vi "Edit Poll.vi"(8 "error in (no error)":errorcluster, 11 "Node Ptr":u64 format="%.0x") -> (0 "error out":errorcluster)   [LabVIEW 2019, in "Diagnostics Addon System Explorer.lvlib"]
uses:
  Diagnostics Addon System Explorer.lvlib
  <vilib>/NI VeriStand/Custom Device Tools/Custom Device Utility Library/Custom Device Utility Library.lvlib
  Types/FG.Action.ctl
  <vilib>/NI VeriStand/Custom Device API/Custom Device API.lvlib
  Types/Poll.LinkedNode.ctl
panel:
  in  "Tag":string
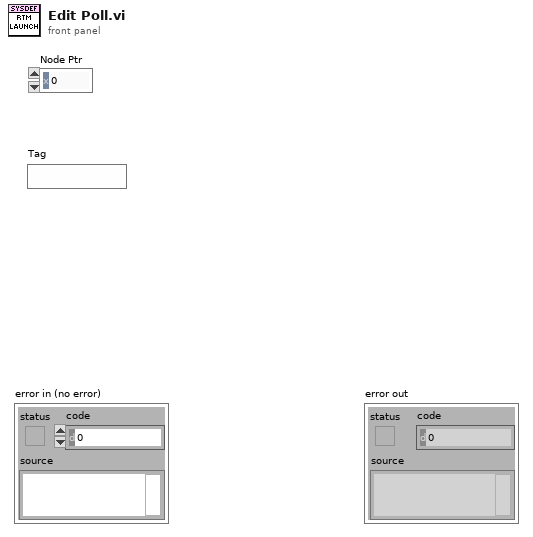
[diagram p1: front panel]
types:
  T1 = typedef "Diagnostics Addon System Explorer.lvlib/Poll.LinkedNode.ctl" = cluster{"Node ID":u64}
  T2 = typedef "Diagnostics Addon System Explorer.lvlib/FG.Action.ctl" = enum16{"Get", "Set"}
  T3 = typedef "Custom Device API.lvlib/Custom Device Item Ref.ctl" = u64
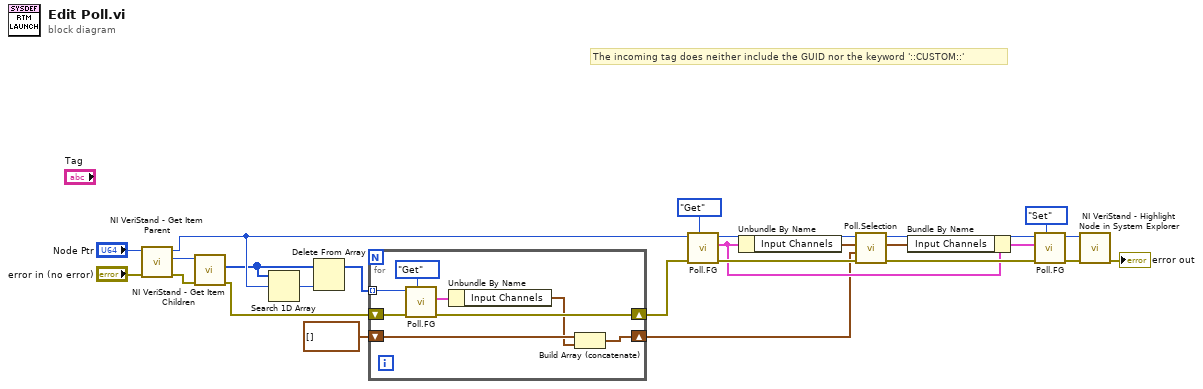
[diagram p0: block diagram]
diagram:
  # "The incoming tag does neither include the GUID nor the keyword '::CUSTOM::'"
  n1 = call <vilib>:"NI VeriStand - Get Item Parent.vi"("error in (no error)"="error in (no error)", "Item Ref in"="Node Ptr") -> ("error out"=w12:errorcluster, "Parent Ref"=w11:T3, "Item Ref out"=w8:T3)  [unwired: 6 in, 1 out]
  n2 = call <vilib>:"NI VeriStand - Get Item Children.vi"("error in (no error)"=w12, "Item Ref in"=w11) -> ("error out"=w4:errorcluster, "Child Refs"=w6:T3[])  [unwired: 6 in, 2 out]
  n3 = Search 1D Array(1D array=w6, element=w8) -> (index of element=w7:i32)  [unwired: 1 in]
  n4 = Delete From Array(array=w6, index=w7) -> (array with subset deleted=w5:T3[])  [unwired: 1 in, 1 out]
  n5 = for {
    tunnel: w5 -> [w31] mode=indexing
    shift-right: [w29] -> w2
    shift-left: w4 -> [w30]
    shift-right: [w26] -> w1
    shift-left: T1[] [] ("Input Channels") -> [w28]
    n6 = call "Poll.FG.vi"("Action"=FG.Action."Get", "error in"=w30, "Parent Ref"=w31) -> ("error out"=w29:errorcluster, "Selected Channels out"=w33:cluster{"Input Channels":T1[]})  [unwired: 6 in, 1 out]
    n7 = Unbundle By Name(w33) -> ("Input Channels"=w27:T1[])
    n8 = Build Array (concatenate)(w28, w27) -> (w26:T1[])
  }
  n9 = call "Poll.FG.vi"("Action"=FG.Action."Get", "error in"=w2, "Parent Ref"=w8) -> ("error out"=w22:errorcluster, "Selected Channels out"=w18:cluster{"Input Channels":T1[]}, "Parent Ref Out"=w23:T3)  [unwired: 6 in]
  n10 = Unbundle By Name(w18) -> ("Input Channels"=w21:T1[])
  n11 = call "Poll.Selection.vi"("error in (no error)"=w22, "Already Used"=w1, "Input Channels"=w21, "Node Ptr"=w23) -> ("error out"=w19:errorcluster, "Input Channel Selections"=w17:T1[], "Node Ptr out"=w15:T3)  [unwired: 5 in]
  n12 = Bundle By Name(cluster=w18, "Input Channels"=w17) -> (w16:cluster{"Input Channels":T1[]})
  n13 = call "Poll.FG.vi"("Action"=FG.Action."Set", "error in"=w19, "Selected Channels"=w16, "Parent Ref"=w15) -> ("error out"=w14:errorcluster, "Parent Ref Out"=w13:T3)  [unwired: 5 in, 1 out]
  n14 = call <vilib>:"NI VeriStand - Highlight Node in System Explorer.vi"("error in (no error)"=w14, "Item Ref in"=w13) -> ("error out"=→"error out":errorcluster)  [unwired: 8 in, 1 out]
